vi "maxInRoi.vi"(8 "useROI":bool, 9 "ROI Descriptor":T2 {"Contours"."Type" items=["No Selection", "Point", "Line", "Rectangle", "Oval", "Polygon", "Freehand Region", "Annulus", "Unused2", "Unused3", "Broken Line", "Freehand Line", "Rotated Rectangle"]}, 11 "Image":T1) -> (0 "max (ROI)":i16, 1 "mean (ROI)":dbl, 3 "Image Out":T1)   [LabVIEW 2017]
uses:
  <vilib>/vision/Image Controls.llb/IMAQ Image.ctl
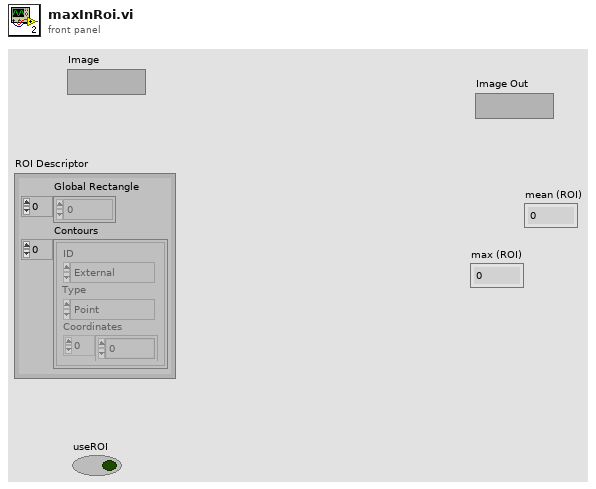
[diagram p1: front panel]
types:
  T1 = typedef "IMAQ Image.ctl" = refnum<image>
  T2 = cluster{"Global Rectangle":i32[], "Contours":cluster{"ID":enum32{"External", "Internal"}, "Type":u32, "Coordinates":i32[]}[]}
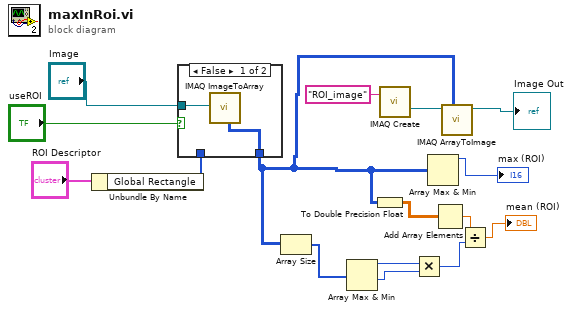
[diagram p0: block diagram]
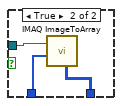
[diagram p2: hidden frame]
diagram:
  n1 = Unbundle By Name("ROI Descriptor") -> ("Global Rectangle"=w16:i32[])
  n2 = case shown="False" "useROI" {
    tunnel: [w17 w21] -> w3
    tunnel: w16 -> [_ w19]
    tunnel: "Image" -> [w18 w20]
    frame False {
      n3 = call "IMAQ ImageToArray"("Image"=w18) -> ("Image Pixels (U16)"=w17:u16[][])  [unwired: 3 in, 4 out]
    }
    frame True {
      n4 = call "IMAQ ImageToArray"("Optional Rectangle"=w19, "Image"=w20) -> ("Image Pixels (U16)"=w21:u16[][])  [unwired: 2 in, 4 out]
    }
  }
  n5 = Array Size(array=w3) -> (size(s)=w7:i32[])
  n6 = Array Max & Min(array=w7) -> (max value=w6:i32, min value=w1:i32)  [unwired: 2 out]
  n7 = To Double Precision Float(number=w3) -> (double precision float=w2:dbl[][])
  n8 = call "IMAQ Create"("Image Name"="ROI_image") -> ("New Image"=w13:T1)  [unwired: 4 in, 1 out]
  n9 = Multiply(x=w6, y=w1) -> (x*y=w5:i32)
  n10 = Array Max & Min(array=w3) -> (max value=→"max (ROI)":u16)  [unwired: 3 out]
  n11 = Add Array Elements(numeric array=w2) -> (sum=w8:dbl)
  n12 = call "IMAQ ArrayToImage"("Image Pixels (U16)"=w3, "Image"=w13) -> ("Image Out"=→"Image Out":T1)  [unwired: 8 in, 1 out]
  n13 = Divide(x=w8, y=w5) -> (x/y=→"mean (ROI)":dbl)
